vi "Read Data.vi"(8 "error in (no error)":errorcluster, 10 "COMMAND":string, 11 "VISA resource name in":refnum<visa-resource-name>) -> (0 "error out":errorcluster, 2 "Output":string, 3 "VISA resource name out":refnum<visa-resource-name>)   [LabVIEW 2010, in "DPR250.lvlib"]
uses:
  DPR250.lvlib
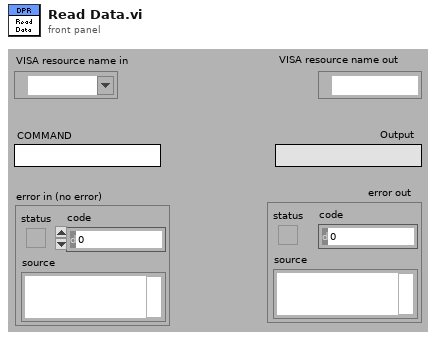
[diagram p1: front panel]
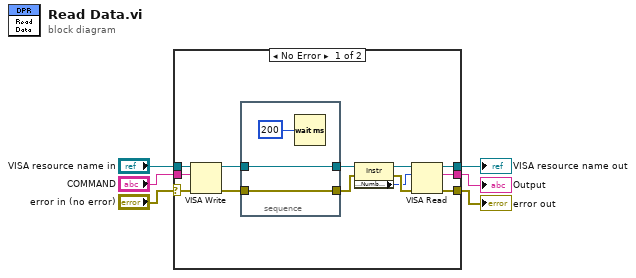
[diagram p0: block diagram]
diagram:
  n1 = case shown="No Error" "error in (no error)" {
    selector: "error in (no error)" -> [w8 w23]
    tunnel: "COMMAND" -> [w19 _]
    tunnel: "VISA resource name in" -> [w18 w24]
    tunnel: [w11 w24] -> w4
    tunnel: [w10 w23] -> w3
    tunnel: [w9 _] -> w2
    frame No Error {
      n2 = VISA Write(VISA resource name=w18, write buffer=w19, error in (no error)=w8) -> (VISA resource name out=w15:refnum<visa-resource-name>, error out=w17:errorcluster)  [unwired: 1 out]
      n3 = stacked-sequence {
        tunnel: w17 -> [w22]
        tunnel: [w22] -> w16
        tunnel: w15 -> [w21]
        tunnel: [w21] -> w14
        frame #0 {
          n4 = Wait (ms)(milliseconds to wait=u32 200 ("delay read (ms)")) -> ()  [unwired: 1 out]
        }
      }
      n5 = property class="Instr"(reference=w14, error in=w16) -> (reference out=w13:refnum<visa-resource-name>, error out=w12:errorcluster, "Serial Settings:Number of Bytes at Serial Port"=w7:u32)
      n6 = VISA Read(VISA resource name=w13, byte count=w7, error in (no error)=w12) -> (VISA resource name out=w11:refnum<visa-resource-name>, read buffer=w9:string, error out=w10:errorcluster)  [unwired: 1 out]
    }
    frame Error {
    }
  }
  "error out" <- w3
  "VISA resource name out" <- w4
  "Output" <- w2
